vi "Secured MQTT Publisher for Labview.vi"() -> ()   [LabVIEW 2021]
uses:
  <vilib>/LabVIEW Open Source Project/MQTT Client/Client class/Client.lvclass
  C:/Program Files (x86)/National Instruments/LabVIEW 2021/vi.lib/LabVIEW Open Source Project/MQTT Connection/MQTT_Base/Base Class/MQTT_Base.lvclass
  <vilib>/LabVIEW Open Source Project/MQTT Connection/MQTT_Base/Base Class/MQTT_Base.lvclass
  <vilib>/LabVIEW Open Source Project/MQTT Secured TCP Connection/Connection.SecuredTCP/Connection.TCP-TLS.lvclass
panel:
  in  "Hostname":string="mqtt.favoriot.com"
  in  "address (localhost)":string="mqtt.favoriot.com"
  in  "Server X.509 Certificate crt":path
  out "Ready for SSL":bool
  in  "Client X.509 Certificate der":path
  in  "Username/Password":string
  in  "Topic Name":string
  in  "Payload Full":string
  out "connected":bool
  out "Published":bool
  out "last error":errorcluster
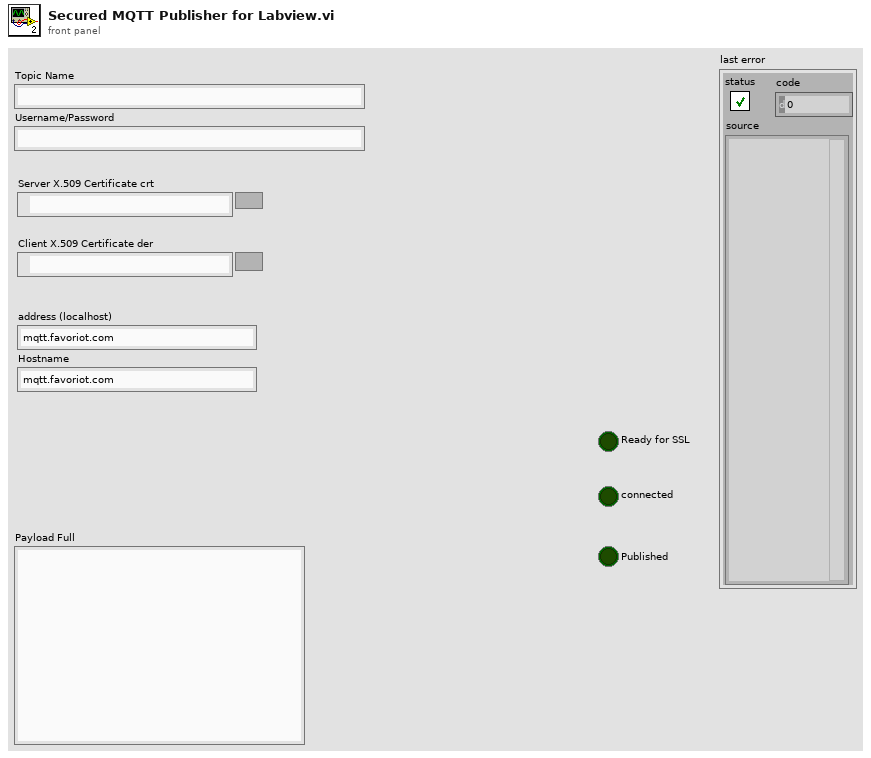
[diagram p1: front panel]
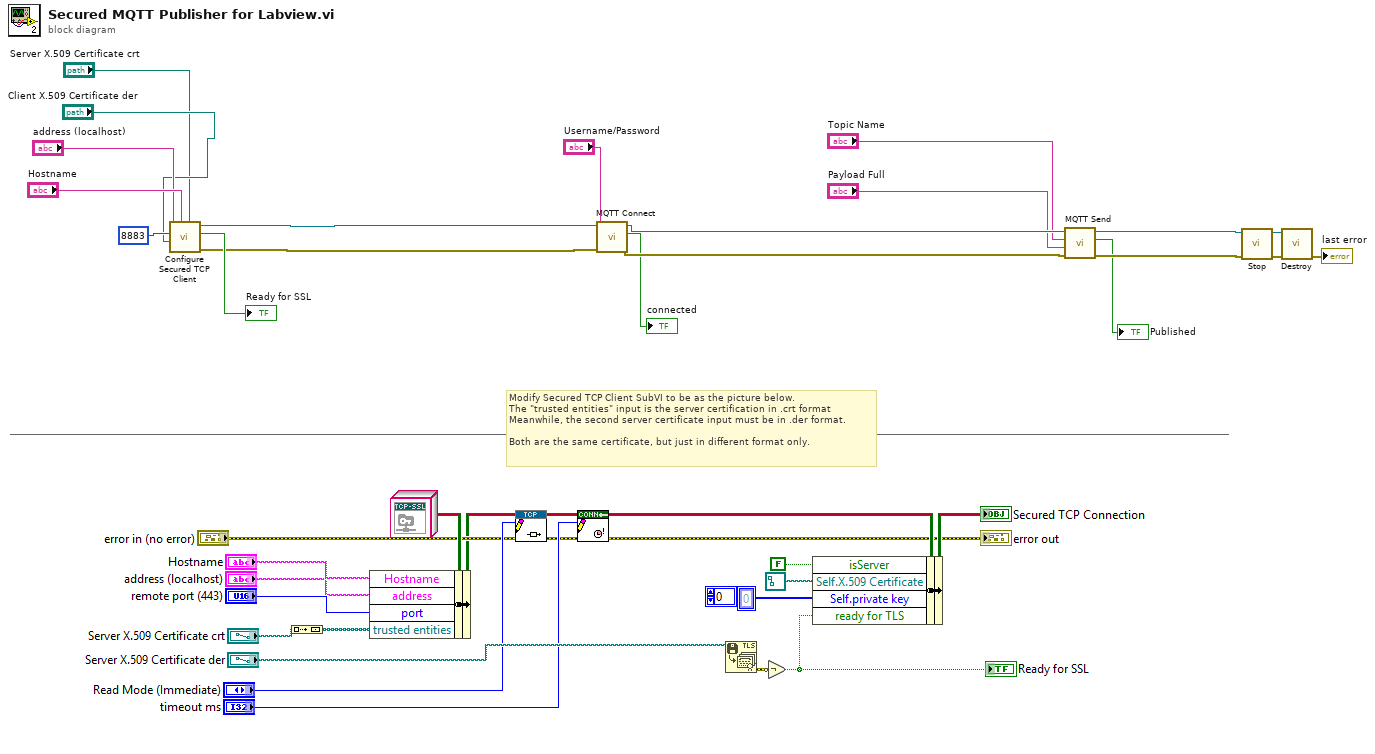
[diagram p0: block diagram]
diagram:
  # "Modify Secured TCP Client SubVI to be as the picture below. \nThe \"trusted entities\" input is the server certification in .crt format\nMeanwhile, the second server certificate input must be in .der format.\n\nBoth are the same certificate, but just in different format only."
  n1 = call <vilib>:"Configure Secured TCP Client.vi"("Server X.509 Certificate crt"="Server X.509 Certificate crt", "Hostname"="Hostname", "Server X.509 Certificate der"="Client X.509 Certificate der", "remote port (443)"=u16 8883 ("remote port (80)"), "address (localhost)"="address (localhost)") -> ("error out"=w1:errorcluster, "Ready for SSL"=→"Ready for SSL":bool, "Secured TCP Connection"=w2:refnum<class "Connection.TCP-TLS.lvclass">)  [unwired: 4 in]
  n2 = call "MQTT Connect.vi"("error in (no error)"=w1, "Username/Password"="Username/Password", "Secured TCP Connection"=w2) -> ("error out"=w14:errorcluster, "connected"=→"connected":bool, "Client out"=w15:refnum<class "Client.lvclass">)  [unwired: 6 in]
  n3 = call "MQTT Send.vi"("error in (no error)"=w14, "Payload Full"="Payload Full", "Topic Name"="Topic Name", "Client in"=w15) -> ("error out"=w19:errorcluster, "Published"=→"Published":bool, "Client out"=w17:refnum<class "Client.lvclass">)  [unwired: 5 in]
  n4 = call <vilib>:"Stop.vi"("error in (no error)"=w19, "MQTT_Base in"=w17) -> ("error out"=w18:errorcluster, "MQTT_Base out"=w16:refnum<class "Client.lvclass">)  [unwired: 7 in, 1 out]
  n5 = call <vilib>:"Destroy.vi"("error in (no error)"=w18, "MQTT_Base in"=w16) -> ("error out"=→"last error":errorcluster)  [unwired: 8 in, 1 out]
